vi "PeriodicFilter-Is String Filtered.vi"(10 "Input String":string, 11 "data in":T1 {"LastCheckT" format="%<%.3X>T"}) -> (0 "Filtered":bool, 2 "Input String (dup)":string, 3 "data out":T1 {"LastCheckT" format="%<%.3X>T"})   [LabVIEW 2017, in "Communicable State Machine.lvlib"]
uses:
  Communicable State Machine.lvlib
  Periodic String Filter Data.ctl
  Periodic String Filter Info.ctl
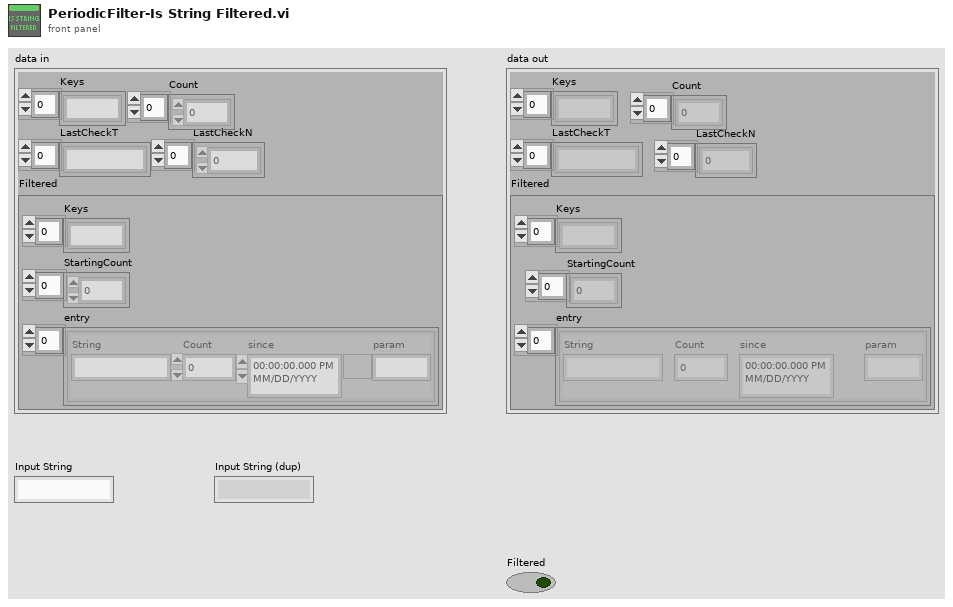
[diagram p1: front panel]
types:
  T1 = typedef "Communicable State Machine.lvlib/Periodic String Filter Data.ctl" = cluster{"Keys":string[], "Count":i64[], "LastCheckT":timestamp[], "LastCheckN":i64[], "Filtered":cluster{"Keys":string[], "StartingCount":i64[], "entry":T2[]}}
  T2 = typedef "Communicable State Machine.lvlib/Periodic String Filter Info.ctl" = cluster{"String":string, "Count":i64, "since":timestamp, "param":string}
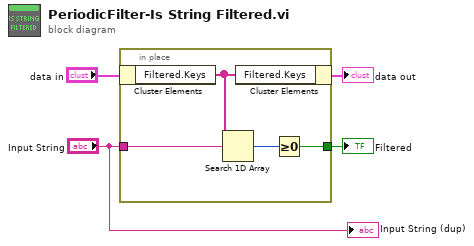
[diagram p0: block diagram]
diagram:
  n1 = in-place "In Place Element Structure" {
    in-place-border: "Input String" -> [w7]
    in-place-border: [w5] -> w4
    n2 = in-place-cluster #1("data in") -> ("Filtered.Keys"=w8:string[])
    n3 = Search 1D Array(1D array=w8, element=w7) -> (index of element=w6:i32)  [unwired: 1 in]
    n4 = in-place-cluster #1("Filtered.Keys"=w8) -> (→"data out":T1)
    n5 = Greater Or Equal To 0?(x=w6) -> (x >= 0?=w5:bool)
  }
  "Filtered" <- w4
  "Input String (dup)" <- "Input String"
